vi "json_parse_number.vi"(8 "error in (no error)":errorcluster, 11 "data":string) -> (0 "error out":errorcluster, 2 "value":variant, 3 "remaining data":string)   [LabVIEW 2017]
uses:
  <vilib>/regexp/Match Regular Expression.xnode
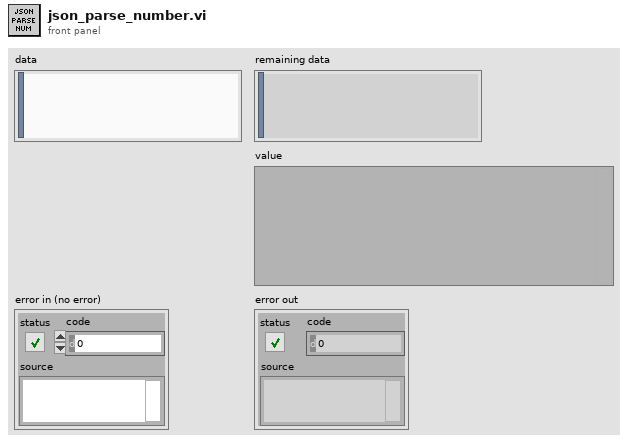
[diagram p1: front panel]
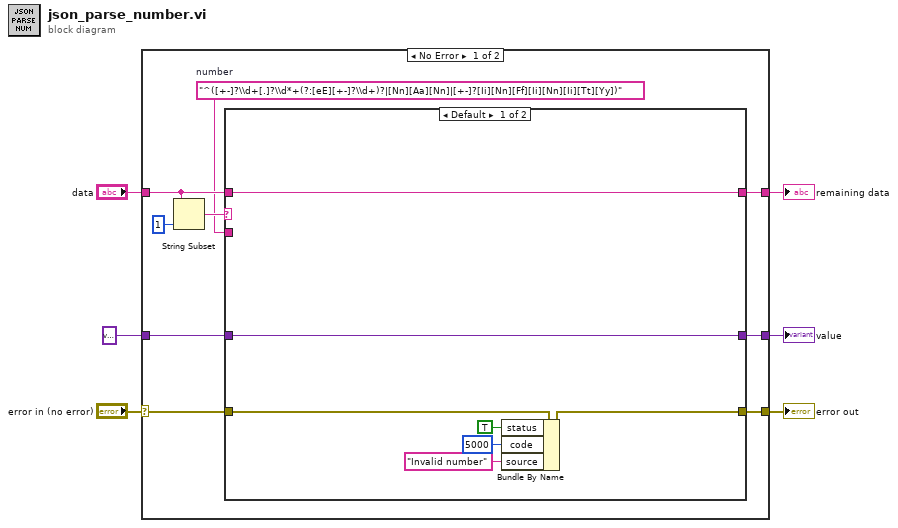
[diagram p0: block diagram]
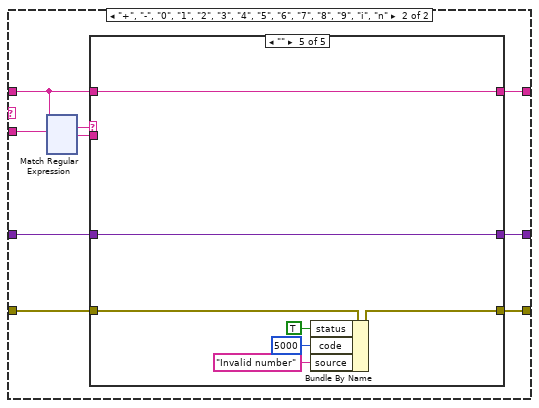
[diagram p2: hidden frame]
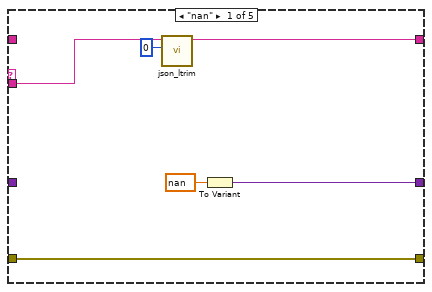
[diagram p3: hidden frame]
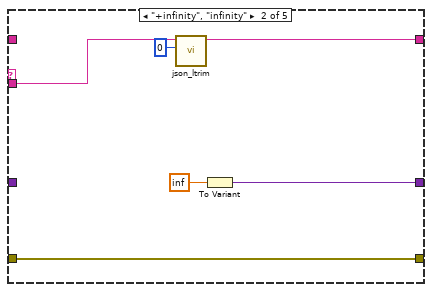
[diagram p4: hidden frame]
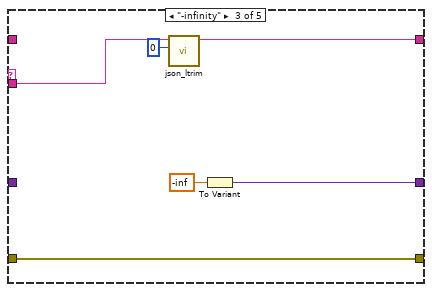
[diagram p5: hidden frame]
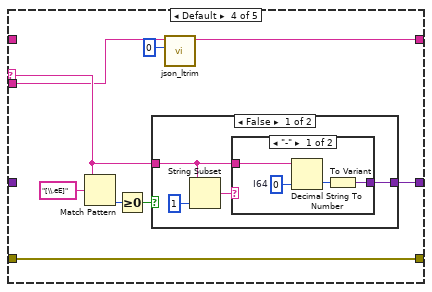
[diagram p6: hidden frame]
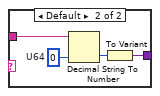
[diagram p7: hidden frame]
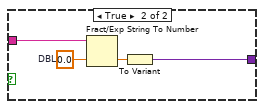
[diagram p8: hidden frame]
diagram:
  n1 = case shown="No Error" "error in (no error)" {
    selector: "error in (no error)" -> [w9 w198]
    tunnel: [w15 w196] -> w6
    tunnel: [w14 w197] -> w5
    tunnel: "data" -> [w13 w197]
    tunnel: [w10 w198] -> w3
    tunnel: variant ("Variant") -> [w7 w196]
    frame No Error {
      w8 = "^([+-]?\\d+[.]?\\d*+(?:[eE][+-]?\\d+)?|[Nn][Aa][Nn]|[+-]?[Ii][Nn][Ff][Ii][Nn][Ii][Tt][Yy])"  # number
      n2 = String Subset(string=w13, length (rest)=1 ("length (rest)")) -> (substring=w11:string)  [unwired: 1 in]
      n3 = case shown="Default" w11 {
        tunnel: w13 -> [w21 w24]
        tunnel: [w22 w29] -> w15
        tunnel: w7 -> [w22 w23]
        tunnel: [w21 w31] -> w14
        tunnel: [w19 w26] -> w10
        tunnel: w9 -> [w20 w25]
        tunnel: w8 -> [_ w30]
        frame Default {
          n4 = Bundle By Name(cluster=w20, "status"=TRUE, "code"=5000, "source"="Invalid number") -> (w19:errorcluster)
        }
        frame "+", "-", "0", "1", "2", "3", "4", "5", "6", "7", "8", "9", "i", "n" {
          n5 = xnode "Match Regular Expression"("input string"=w24, "regular expression"=w30) -> ("whole match"=w27:string, "after match"=w28:string)  [unwired: 4 in, 3 out]
          n6 = case shown="\"\"" w27 {
            selector: w27 -> [_ _ _ w55 _]
            tunnel: [w33 w38 w44 w50 w81] -> w31
            tunnel: [w36 w42 w48 w58 w75] -> w29
            tunnel: w28 -> [w34 w39 w45 w51 _]
            tunnel: [w35 w41 w47 w53 w76] -> w26
            tunnel: w25 -> [w35 w41 w47 w53 w77]
            tunnel: w24 -> [_ _ _ _ w81]
            tunnel: w23 -> [_ _ _ _ w75]
            frame "nan" {
              n7 = call "json_ltrim.vi"("offset (0)"=0, "data"=w34) -> ("left trim whitespace"=w33:string)  [unwired: 9 in]
              n8 = To Variant(anything=nan) -> (Variant=w36:variant)
            }
            frame "+infinity", "infinity" {
              n9 = call "json_ltrim.vi"("offset (0)"=0, "data"=w39) -> ("left trim whitespace"=w38:string)  [unwired: 9 in]
              n10 = To Variant(anything=inf) -> (Variant=w42:variant)
            }
            frame "-infinity" {
              n11 = call "json_ltrim.vi"("offset (0)"=0, "data"=w45) -> ("left trim whitespace"=w44:string)  [unwired: 9 in]
              n12 = To Variant(anything=-inf) -> (Variant=w48:variant)
            }
            frame Default {
              n13 = Match Pattern(string=w55, regular expression="[\\.eE]") -> (offset past match=w56:i32)  [unwired: 1 in, 3 out]
              n14 = Greater Or Equal To 0?(x=w56) -> (x >= 0?=w54:bool)
              n15 = case shown="False" w54 {
                tunnel: w55 -> [w61 w74]
                tunnel: [w60 w71] -> w58
                frame False {
                  n16 = String Subset(string=w61, length (rest)=1 ("length (rest)")) -> (substring=w59:string)  [unwired: 1 in]
                  n17 = case shown="\"-\"" w59 {
                    tunnel: w61 -> [w66 w70]
                    tunnel: [w63 w67] -> w60
                    frame "-" {
                      w65 = i64 0  # I64
                      n18 = Decimal String To Number(string=w66, default (0L)=w65) -> (number=w64:i64)  [unwired: 1 in, 1 out]
                      n19 = To Variant(anything=w64) -> (Variant=w63:variant)
                    }
                    frame Default {
                      w69 = u64 0  # U64
                      n20 = Decimal String To Number(string=w70, default (0L)=w69) -> (number=w68:u64)  [unwired: 1 in, 1 out]
                      n21 = To Variant(anything=w68) -> (Variant=w67:variant)
                    }
                  }
                }
                frame True {
                  w73 = 0.0  # DBL
                  n22 = Fract/Exp String To Number(string=w74, default (0 dbl)=w73) -> (number=w72:dbl)  [unwired: 2 in, 1 out]
                  n23 = To Variant(anything=w72) -> (Variant=w71:variant)
                }
              }
              n24 = call "json_ltrim.vi"("offset (0)"=0, "data"=w51) -> ("left trim whitespace"=w50:string)  [unwired: 9 in]
            }
            frame "" {
              n25 = Bundle By Name(cluster=w77, "status"=TRUE, "code"=5000, "source"="Invalid number") -> (w76:errorcluster)
            }
          }
        }
      }
    }
    frame Error {
    }
  }
  "remaining data" <- w5
  "value" <- w6
  "error out" <- w3
